vi "YTO_Read_PLL_Corr_volt_Naoj_2.vi"(5 "Cartridge band":u32 max=10 step=1, 7 "Slave Node in":cluster{"Address":i16, "Serial Number":i8[]}={"Address"=19, "Serial Number"=[16, 71, 55, 76, 1, 8, 0, -15]} {"Serial Number" format="%.0x"; "Address" format="%.0x"}, 8 "error IO":errorcluster, 11 "ObjHandle in":u32) -> (0 "error":errorcluster, 1 "PLL Corr Voltage [V]":sgl, 3 "ObjHandle out":u32, 4 "Lock??":bool)   [LabVIEW 2017]
panel:
  # "Node Address"
  # "Serial Number"
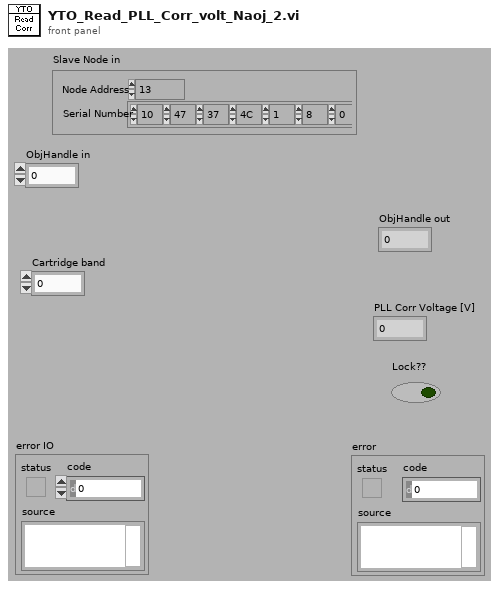
[diagram p1: front panel]
types:
  T1 = cluster{"PLL_ASSY_T":sgl, "PLL_REF_TOT_P":sgl, "PLL_IF_TOT_P":sgl, "PLL_CORR_V":sgl, "PLL_LOCK_V":sgl, "PLL_5V_SUPPLY_V":sgl, "Temp_TF":bool, "PLL Ref Pwr_TF":bool, "IF Pwr_TF":bool, "PLL Corr_TF":bool, "PLL Lock V_TF":bool, "PLL Nominal_TF":bool}
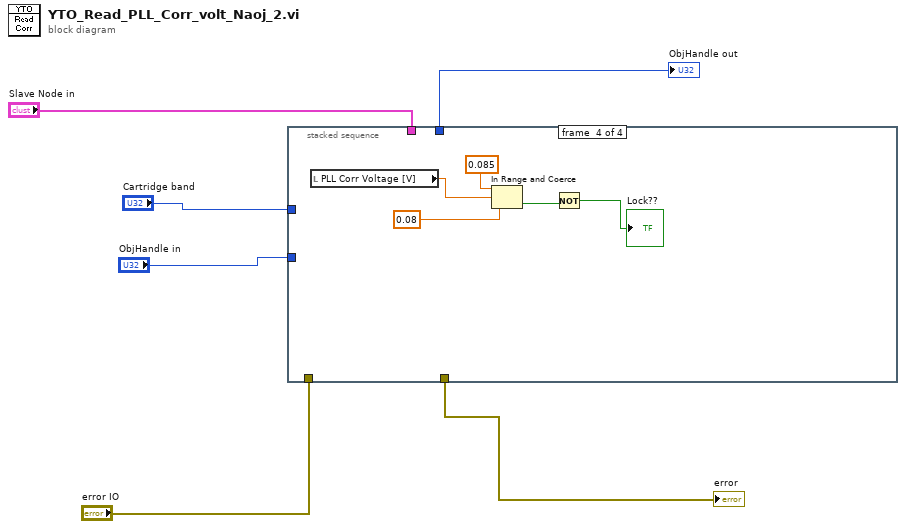
[diagram p0: block diagram]
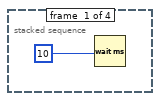
[diagram p2: hidden frame]
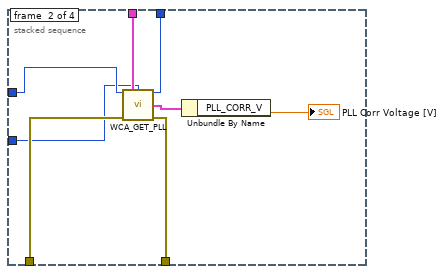
[diagram p3: hidden frame]
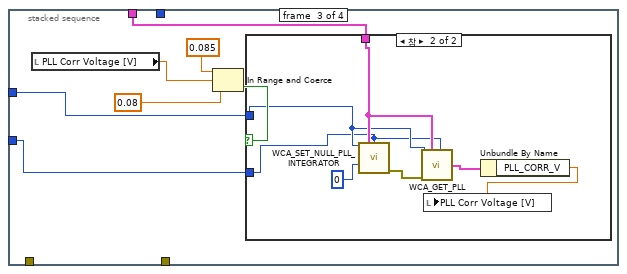
[diagram p4: hidden frame]
diagram:
  n1 = stacked-sequence {
    tunnel: "Slave Node in" -> [_ w14 w16 _]
    tunnel: "ObjHandle in" -> [_ w8 w17 _]
    tunnel: [_ w12 _ _] -> w4
    tunnel: "Cartridge band" -> [_ w9 w18 _]
    tunnel: "error IO" -> [_ w11 _ _]
    tunnel: [_ w10 _ _] -> w1
    frame #0 {
      n2 = Wait (ms)(milliseconds to wait=10) -> ()  [unwired: 1 out]
    }
    frame #1 {
      n3 = call "WCA_GET_PLL.vi"("Cartridge Band"=w9, "Slave Node in"=w14, "ObjHandle in"=w8, "error in (no error)"=w11) -> ("ObjHandle out"=w12:u32, "GET_PLL"=w13:T1, "error out"=w10:errorcluster)  [unwired: 9 in]
      n4 = Unbundle By Name(w13) -> ("PLL_CORR_V"=→"PLL Corr Voltage [V]":sgl)
    }
    frame #2 {
      n5 = local read "PLL Corr Voltage [V]"() -> (w22:sgl)
      n6 = In Range and Coerce(upper limit=0.085, x=w22, lower limit=0.08) -> (In Range?=w19:bool)  [unwired: 1 out]
      n7 = case shown="참" w19 {
        tunnel: w18 -> [_ w24]
        tunnel: w17 -> [_ w23]
        tunnel: w16 -> [_ w26]
        frame False {
        }
        frame True {
          n8 = call "WCA_SET_NULL_PLL_INTEGRATOR.vi"("Cartridge Band"=w24, "Slave Node in"=w26, "ObjHandle in"=w23, "SET_NULL_PLL_INTEGRATOR"=0 ("SET NULL PLL INTEGRATOR")) -> ("error out"=w27:errorcluster)  [unwired: 10 in, 1 out]
          n9 = call "WCA_GET_PLL.vi"("Cartridge Band"=w24, "Slave Node in"=w26, "ObjHandle in"=w23, "error in (no error)"=w27) -> ("GET_PLL"=w28:T1)  [unwired: 9 in, 2 out]
          n10 = Unbundle By Name(w28) -> ("PLL_CORR_V"=w25:sgl)
          n11 = local write "PLL Corr Voltage [V]"(w25) -> ()
        }
      }
    }
    frame #3 {
      n12 = local read "PLL Corr Voltage [V]"() -> (w34:sgl)
      n13 = In Range and Coerce(upper limit=0.085, x=w34, lower limit=0.08) -> (In Range?=w31:bool)  [unwired: 1 out]
      n14 = Not(x=w31) -> (.not. x?=→"Lock??":bool)
    }
  }
  "error" <- w1
  "ObjHandle out" <- w4
